vi "Wait on Call.vi"(8 "error in":errorcluster, 9 "Timeout (ms)":i32=-1, 11 "ASE Handle":refnum<class "ase.lvclass">) -> (0 "error out":errorcluster, 1 "Timeout":bool, 3 "ASE Handle Duplicate":refnum<class "ase.lvclass">)   [LabVIEW 2020, in "ase.lvlib" / "ase.lvclass"]
doc: "<B>Wait for the executable call to exit with an optional timeout.</B>\n\nThis VI is non-blocking so it will not prevent other operations taking place during the wait.\n\nThis VI generates the following errors:\n-5691000: Internal Library Error. Check Error Message for more details.\n1556: Invalid Handle Supplied"
uses:
  ase.lvclass
  ase.lvclass/ase.ctl
  Error Internal Library Implementation Error.vi
  <vilib>/Utility/error.llb/Error Cluster From Error Code.vi
  serenial.io-ase/ase/serenial.io-ase.32.dll
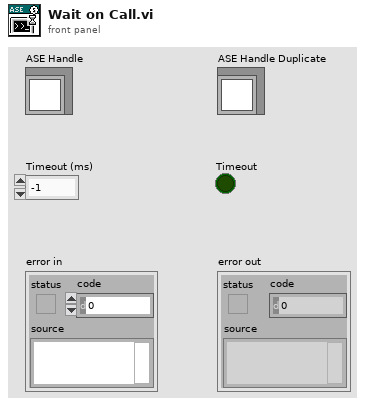
[diagram p1: front panel]
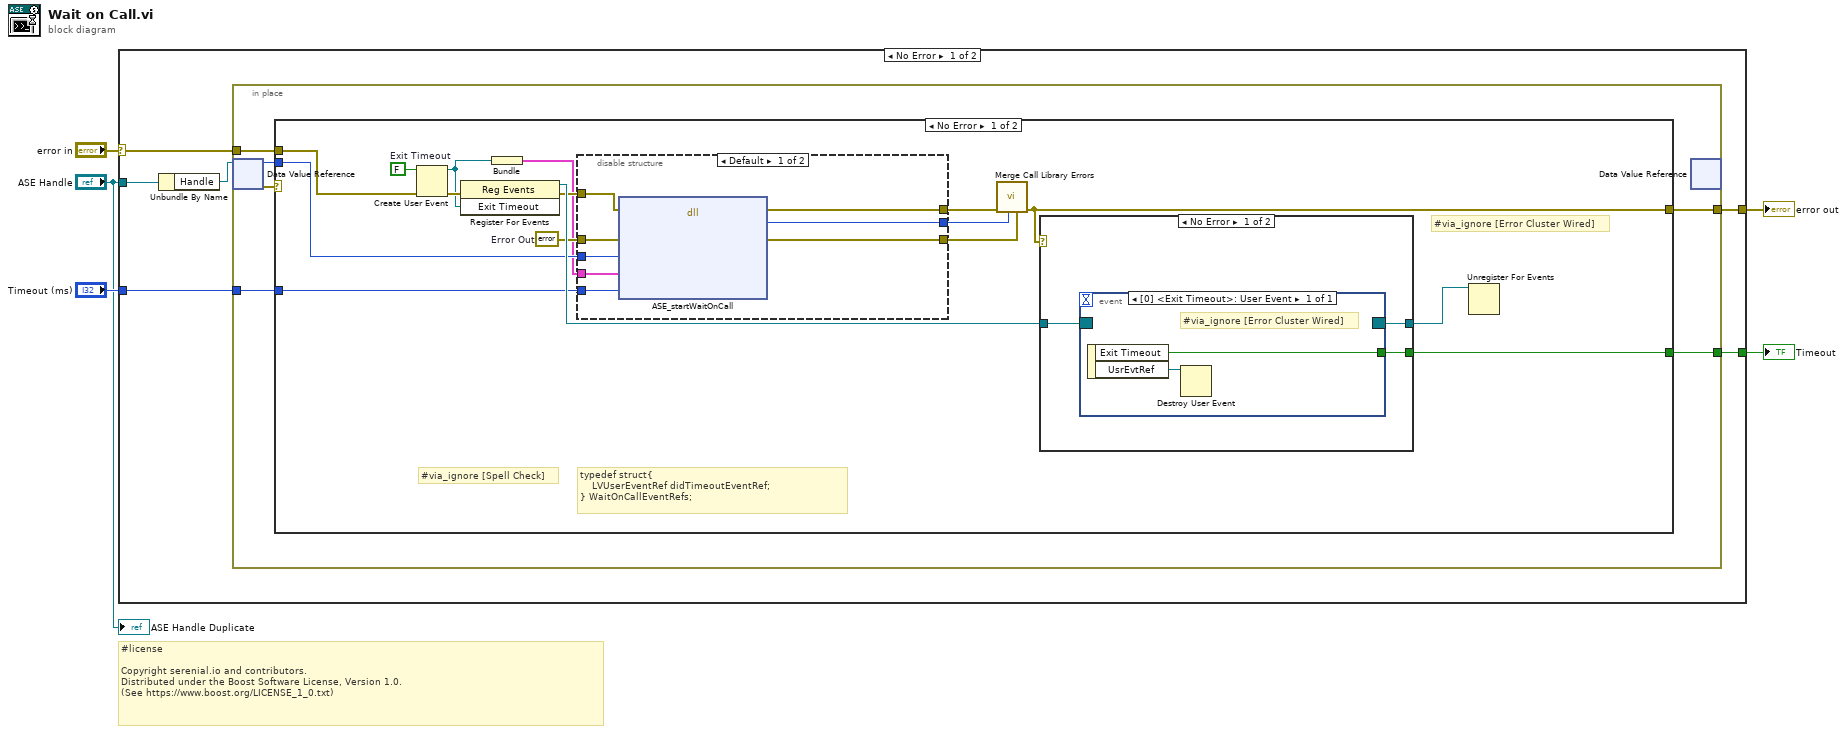
[diagram p0: block diagram]
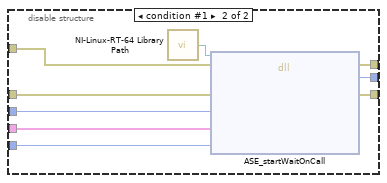
[diagram p2: hidden frame]
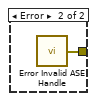
[diagram p4: hidden frame]
diagram:
  # "#license\n\nCopyright serenial.io and contributors.\nDistributed under the Boost Software License, Version 1.0.\n(See https://www.boost.org/LICENSE_1_0.txt)"
  n1 = case shown="No Error" "error in" {
    selector: "error in" -> [w9 w58]
    tunnel: "ASE Handle" -> [w11 _]
    tunnel: "Timeout (ms)" -> [w8 _]
    tunnel: [w7 w58] -> w4
    tunnel: [w6 _] -> w1
    frame No Error {
      n2 = Unbundle By Name(w11) -> ("Handle"=w10:refnum<data-value>)
      n3 = in-place "In Place Element Structure" {
        in-place-border: w9 -> [w15]
        in-place-border: w8 -> [w16]
        in-place-border: [w13] -> w7
        in-place-border: [w12] -> w6
        n4 = in-place-dvr #1 ("Data Value Reference Read / Write Element")(w10) -> (w17:u64, w14:errorcluster)
        n5 = case shown="No Error" w14 {
          tunnel: w17 -> [w23 _]
          tunnel: w16 -> [w21 _]
          tunnel: w15 -> [w33 _]
          tunnel: [w29 w57] -> w13
          tunnel: [w27 _] -> w12
          frame No Error {
            w24 = errorcluster {"status"=FALSE, "code"=0, "source"=""}  # Error Out
            w32 = FALSE  # Exit Timeout
            # "#via_ignore [Error Cluster Wired]"
            # "#via_ignore [Spell Check]"
            # "typedef struct{\n    LVUserEventRef didTimeoutEventRef;\n} WaitOnCallEventRefs;"
            n6 = Create User Event(user event datatype=w32, error in=w33) -> (user event=w30:refnum<user-event>, error out=w31:errorcluster)
            n7 = register-events(error in=w31, w30) -> (reference out=w28:refnum<event-registration>, error out=w25:errorcluster)  [unwired: 1 in]
            n8 = Bundle("Exit Timeout"=w30) -> (w22:cluster{"Exit Timeout":refnum<user-event>})  [unwired: 1 in]
            n9 = disable-structure "Conditional Disable Structure" shown="Default" {
              disable-tunnel: w25 -> [w41 w50]
              disable-tunnel: w24 -> [w40 w49]
              disable-tunnel: w23 -> [w39 w45]
              disable-tunnel: w22 -> [w38 w44]
              disable-tunnel: w21 -> [w37 w43]
              disable-tunnel: [w36 w48] -> w20
              disable-tunnel: [w35 w47] -> w19
              disable-tunnel: [w34 w46] -> w18
              frame condition #0 (active) {
                n10 = dll-call lib="C:/serenial/lib/asynchronous-system-exec/LabVIEW/serenial.io-ase/ase/serenial.io-ase.*.*" fn="ASE_startWaitOnCall" ("serenial.io-ase.32.dll:ASE_writeToStdIn")(error in=w41, "Error Out"=w40, "ASE interface"=w39, "Event Refs"=w38, "Timeout (ms)"=w37) -> (error out=w36:errorcluster, "Error Code"=w35:i32, "Error Out"=w34:errorcluster)  [unwired: 5 in, 1 out]
              }
              frame condition #1 {
                n11 = call "NI-Linux-RT-64 Library Path.vi"() -> ("Path"=w42:path)
                n12 = dll-call lib="?" fn="ASE_startWaitOnCall" ("serenial.io-ase.32.dll:ASE_writeToStdIn")(path in=w42, error in=w50, "Error Out"=w49, "ASE interface"=w45, "Event Refs"=w44, "Timeout (ms)"=w43) -> (error out=w48:errorcluster, "Error Code"=w47:i32, "Error Out"=w46:errorcluster)  [unwired: 4 in, 1 out]
              }
            }
            n13 = call "Merge Call Library Errors.vi"("Library Call Returned Error"=w18, "Error Code"=w19, "error in"=w20) -> ("error IO"=w29:errorcluster)  [unwired: 8 in]
            n14 = case shown="No Error" w29 {
              tunnel: [w53 _] -> w27
              tunnel: w28 -> [w52 w56]
              tunnel: [w51 w56] -> w26
              frame No Error {
                # "Wait for  Thread Wait Timeout Event\n\nDon't lock DVR by waiting inside IPE structure"
                n15 = event shown="[0] <Exit Timeout>: User Event" {
                  selector: w52 -> [_]
                  dyn-events: [_] -> w51
                  timeout: _ -> [_]
                  tunnel: [w55] -> w53
                  event User Event {
                    # "#via_ignore [Error Cluster Wired]"
                    n16 = event-data() -> ("Exit Timeout"=w55:bool, "UsrEvtRef"=w54:refnum<user-event>)  [unwired: 1 in]
                    n17 = Destroy User Event(user event=w54) -> ()  [unwired: 1 in, 1 out]
                  }
                }
              }
              frame Error {
                # "Do Not Wait"
              }
            }
            n18 = Unregister For Events(event registration refnum=w26) -> ()  [unwired: 1 in, 1 out]
          }
          frame Error {
            n19 = call "Error Invalid ASE Handle.vi"() -> ("Invalid ASE Handle"=w57:errorcluster)
          }
        }
        n20 = in-place-dvr #1 ("Data Value Reference Read / Write Element")() -> ()  [unwired: 1 in, 2 out]
      }
    }
    frame Error {
    }
  }
  "error out" <- w4
  "Timeout" <- w1
  "ASE Handle Duplicate" <- "ASE Handle"
